vi "VCNL4010.vi"(8 "i_error":errorcluster, 10 "i_Ref":T1={"Adress"=19, "CMD"=enum."#0 Command Register", "i_Value"=0, "R/W"=enum."Read"} {"i_Value" format="%08b"; "Adress" format="%02x"}) -> (0 "o_error":errorcluster, 2 "o_data":u8 format="%x")   [LabVIEW 2016]
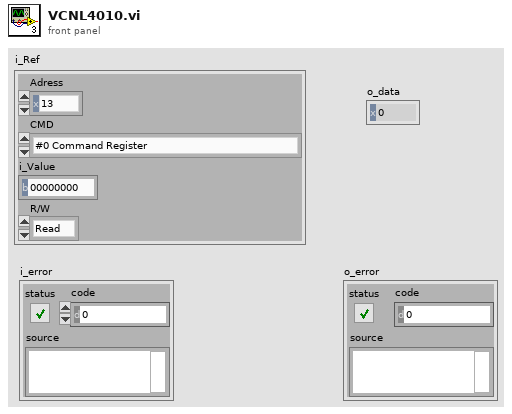
[diagram p1: front panel]
types:
  T1 = cluster{"Adress":u8, "CMD":enum8{"#0 Command Register", "#1 Product ID Revision Register", "#2 Proximity Rate Register", "#3 IR LED Current Register", "#4 Ambient Light Parameter Register", "#5 Ambient Light Result Register", "#6 Ambient Light Result Register", "#7 Proximity Result Register", "#8 Proximity Result Register", "#9 Interrupt Control Register", "#10 Low Threshold Register", "#11 Low Threshold Register", "#12 High Threshold Register", "#13 High Threshold Register", "#14 Interrupt Status Register", "#15 Proximity Modulation Timing Adjustment"}, "i_Value":u8, "R/W":enum16{"Read", "Write"}}
  T2 = enum8{"#0 Command Register", "#1 Product ID Revision Register", "#2 Proximity Rate Register", "#3 IR LED Current Register", "#4 Ambient Light Parameter Register", "#5 Ambient Light Result Register", "#6 Ambient Light Result Register", "#7 Proximity Result Register", "#8 Proximity Result Register", "#9 Interrupt Control Register", "#10 Low Threshold Register", "#11 Low Threshold Register", "#12 High Threshold Register", "#13 High Threshold Register", "#14 Interrupt Status Register", "#15 Proximity Modulation Timing Adjustment"}
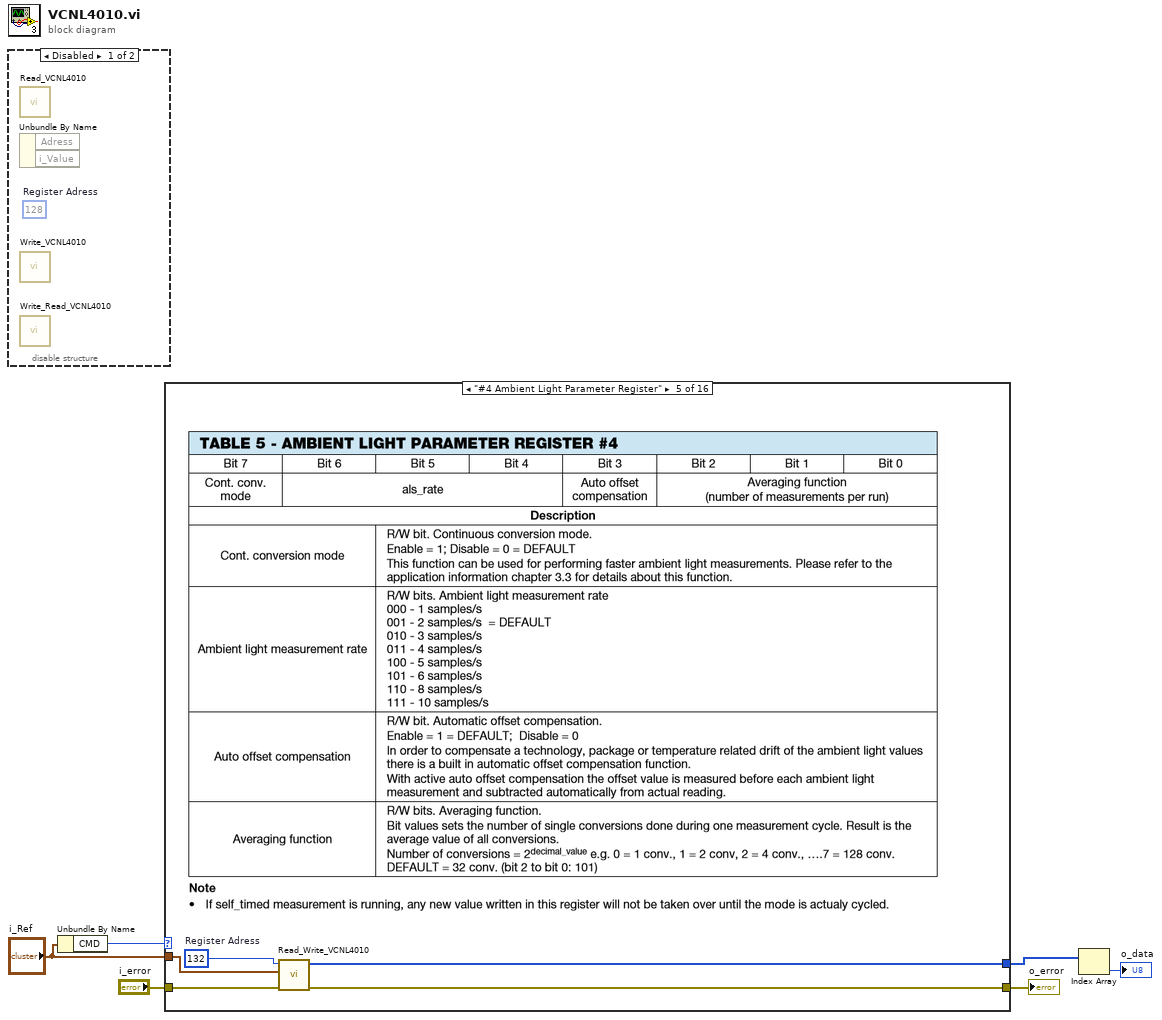
[diagram p0: block diagram]
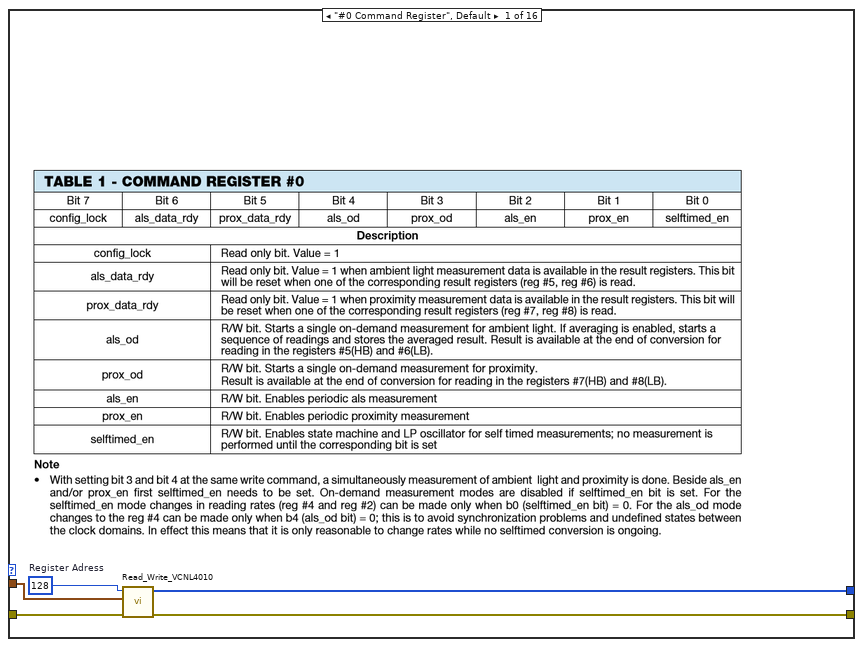
[diagram p2: hidden frame]
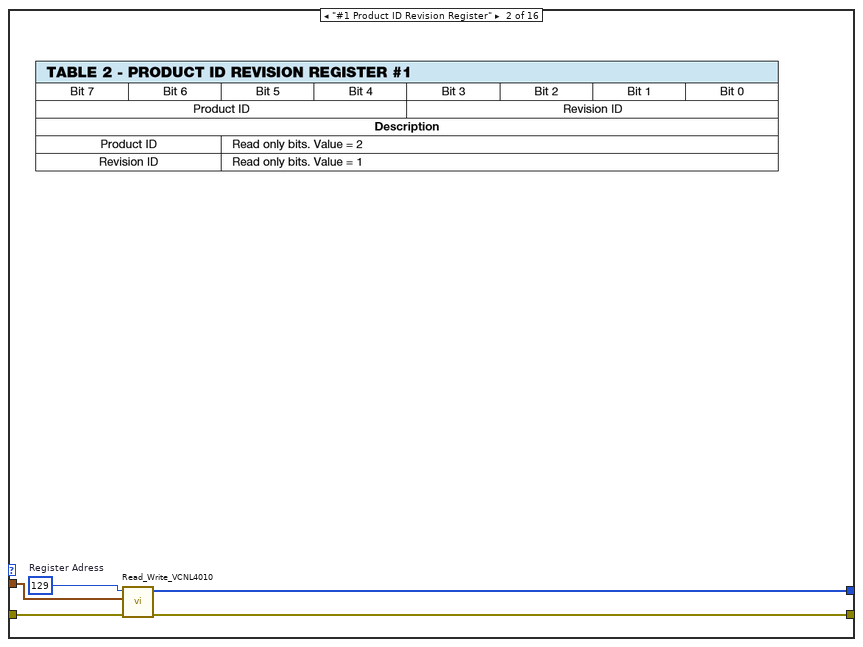
[diagram p3: hidden frame]
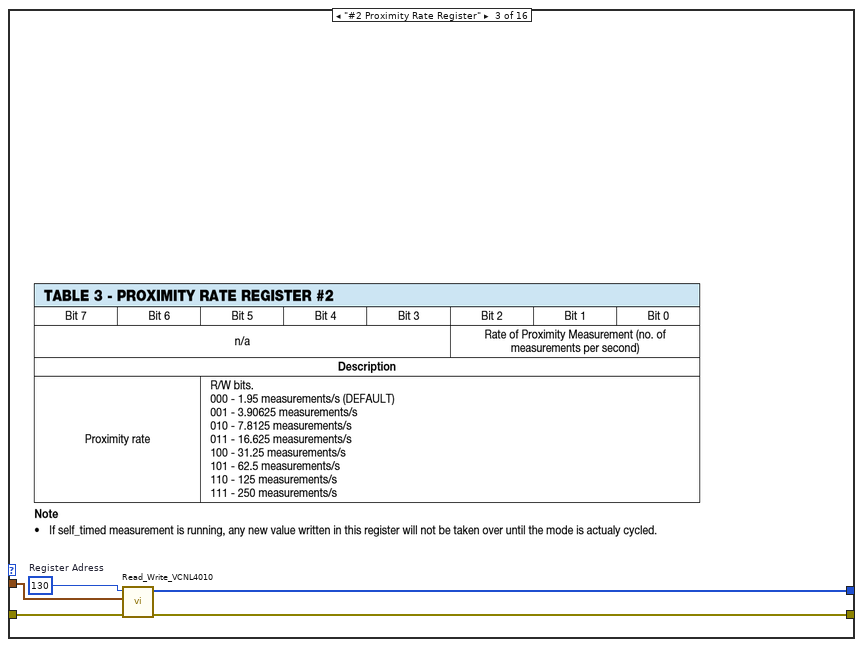
[diagram p4: hidden frame]
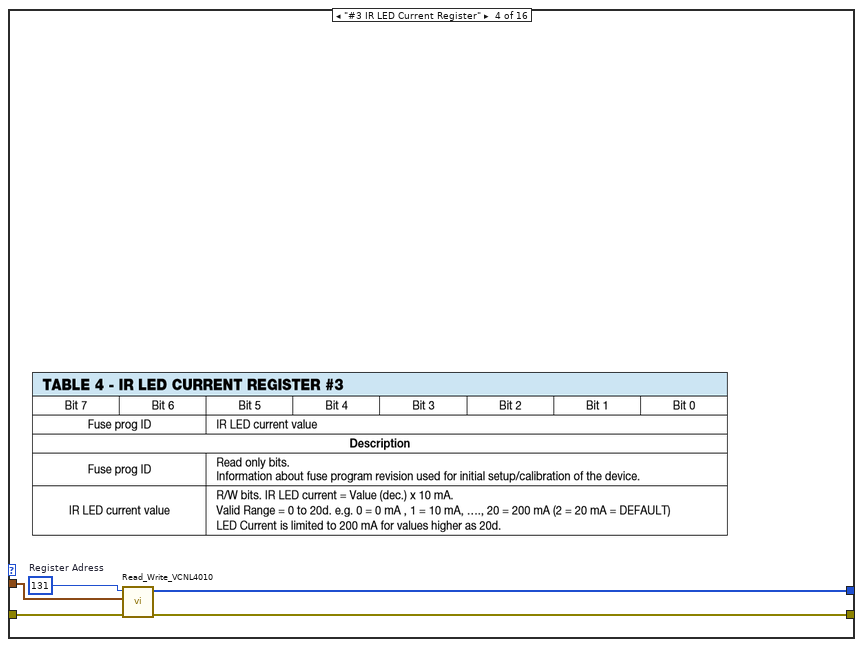
[diagram p5: hidden frame]
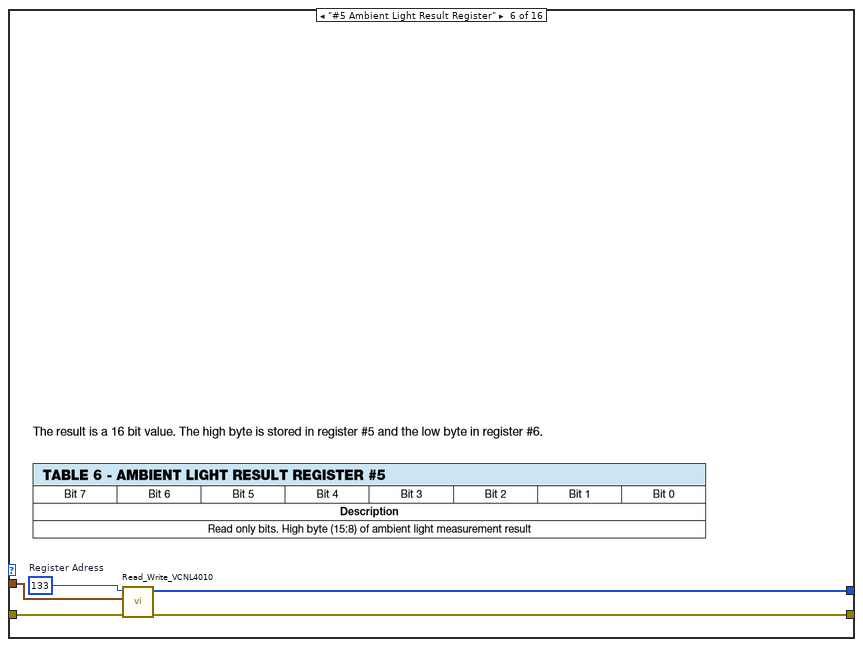
[diagram p6: hidden frame]
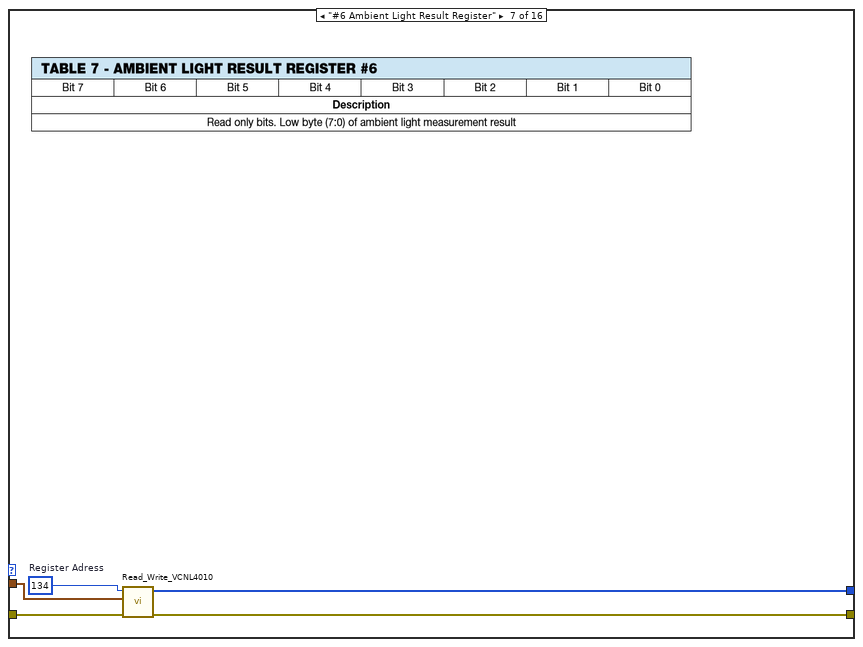
[diagram p7: hidden frame]
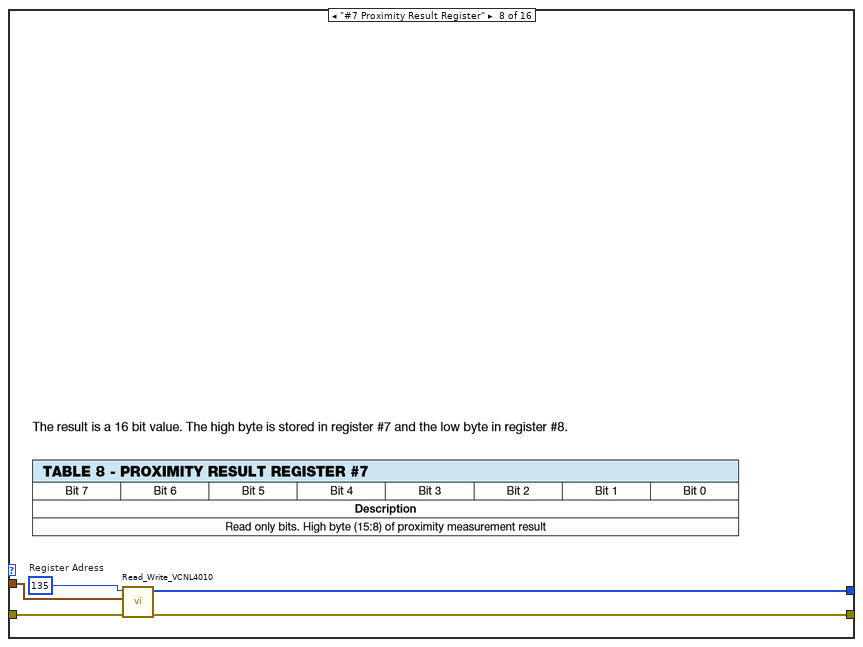
[diagram p8: hidden frame]
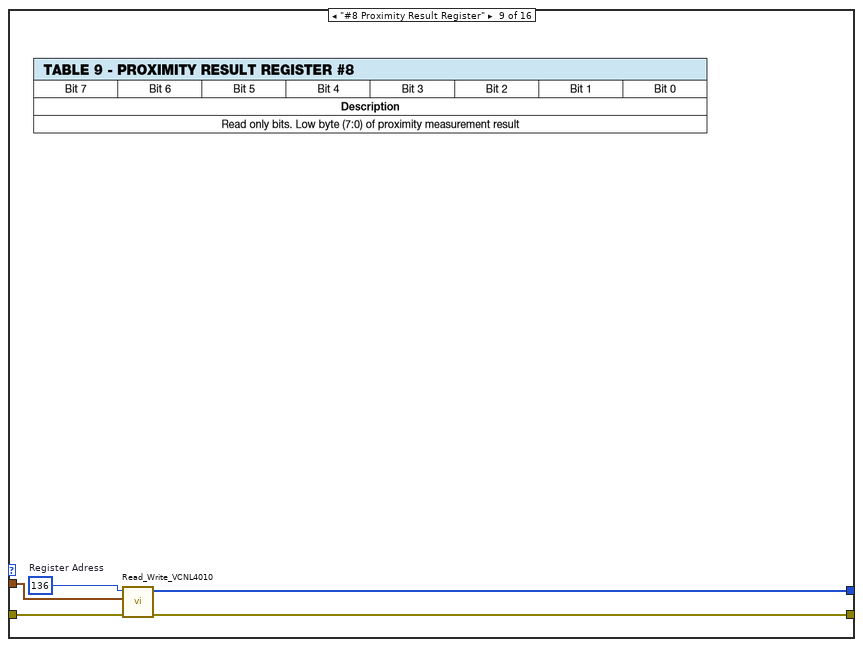
[diagram p9: hidden frame]
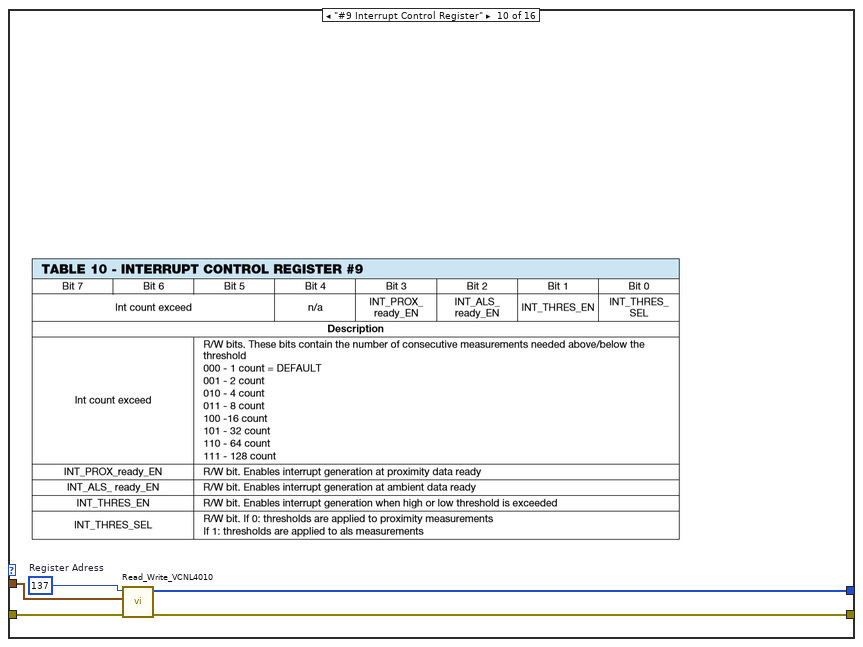
[diagram p10: hidden frame]
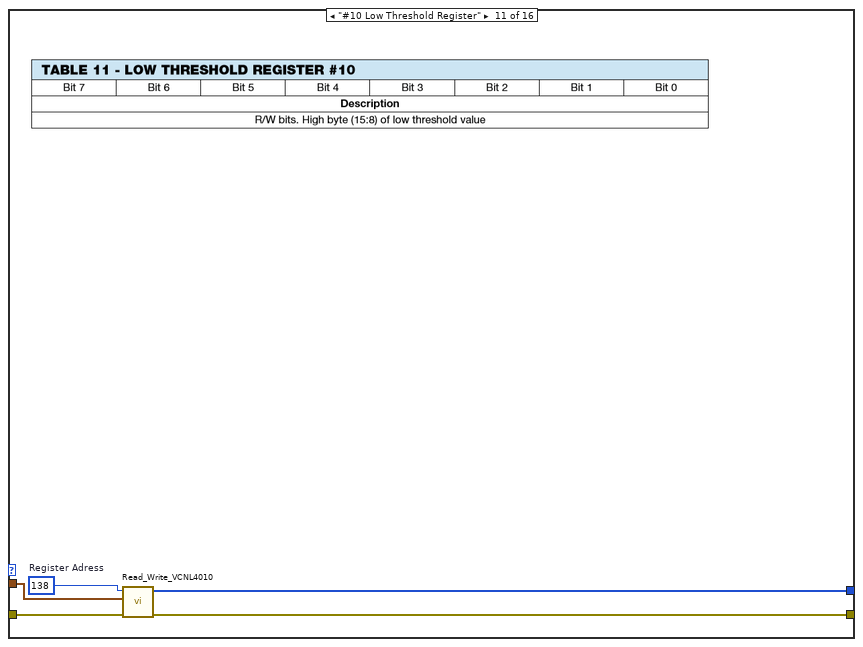
[diagram p11: hidden frame]
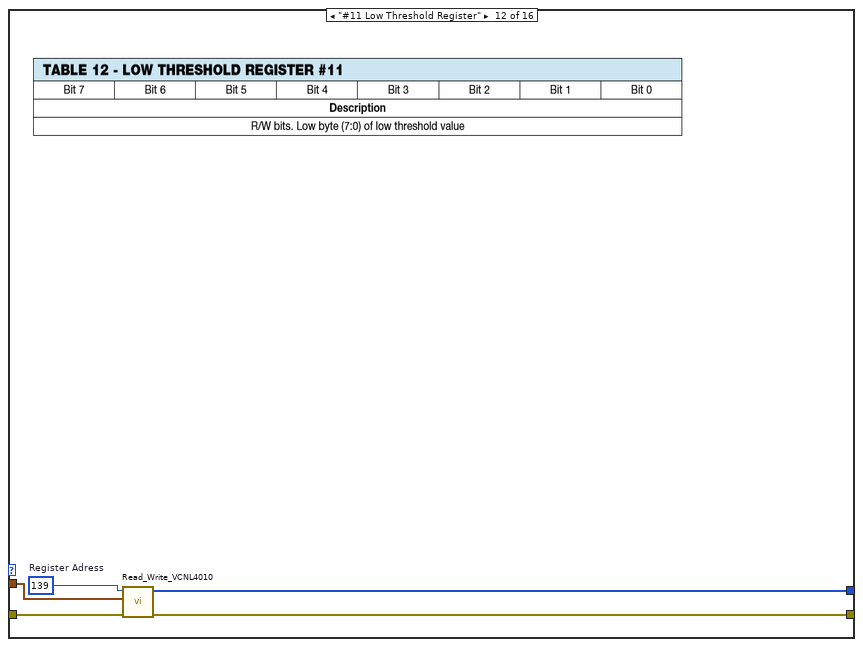
[diagram p12: hidden frame]
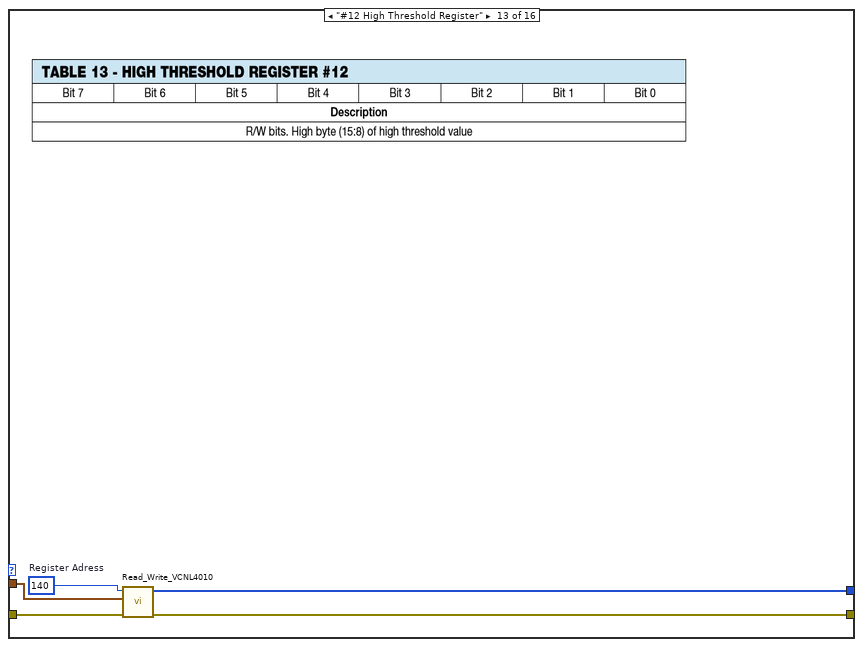
[diagram p13: hidden frame]
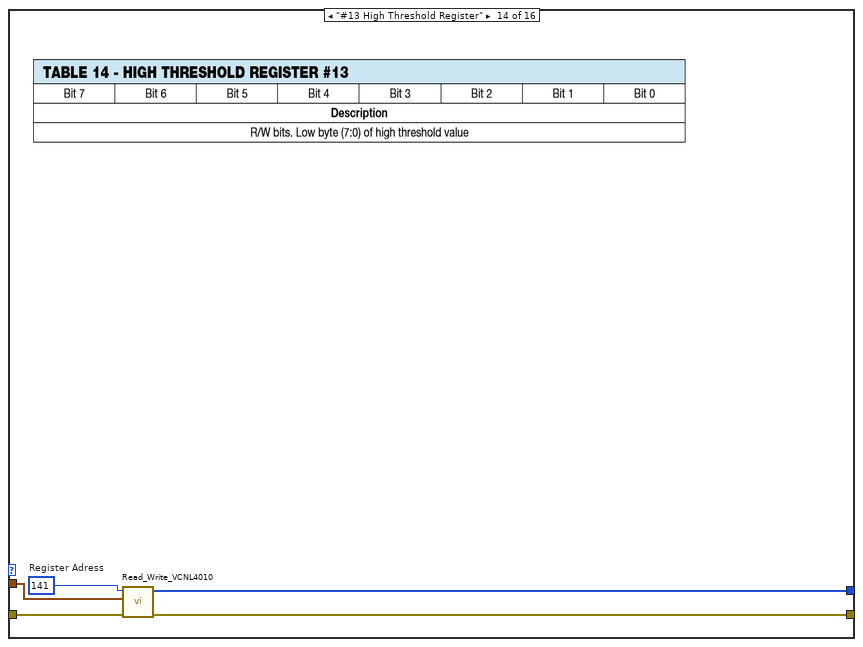
[diagram p14: hidden frame]
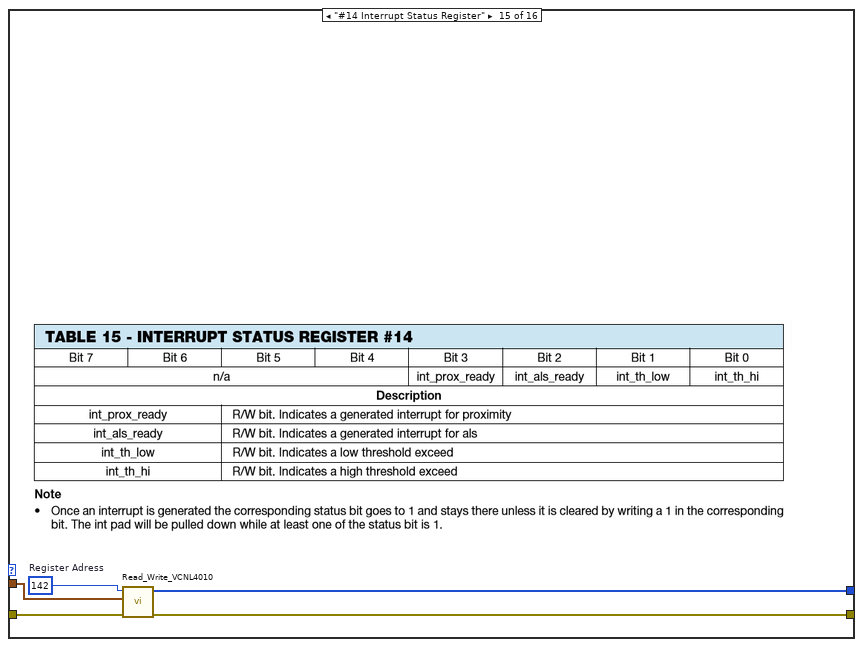
[diagram p15: hidden frame]
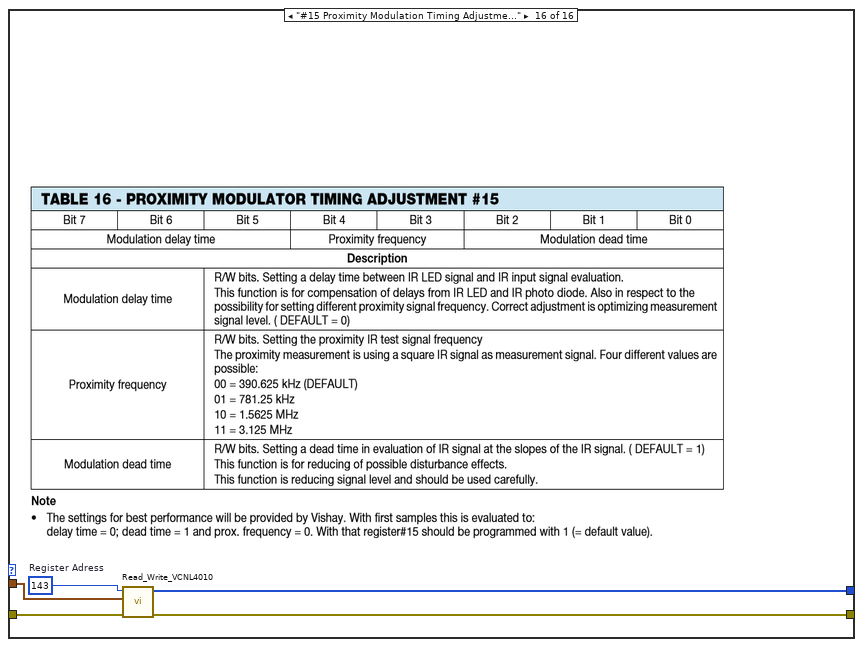
[diagram p16: hidden frame]
diagram:
  n1 = disable-structure shown="Disabled" {
    frame Disabled {
      (unwired) 128  # Register Adress
      n2 = call "Read_VCNL4010.vi"() -> ()  [unwired: 10 in, 2 out]
      n3 = Unbundle By Name() -> ()  [unwired: 1 in, 2 out]
      n4 = call "Write_VCNL4010.vi"() -> ()  [unwired: 11 in, 1 out]
      n5 = call "Write_Read_VCNL4010.vi"() -> ()  [unwired: 10 in, 2 out]
    }
    frame Enabled {
    }
  }
  n6 = Unbundle By Name("i_Ref") -> ("CMD"=w3:T2)
  n7 = case shown="\"#4 Ambient Light Parameter Register\"" w3 {
    tunnel: "i_Ref" -> [w10 w15 w20 w25 w31 w36 w41 w45 w50 w55 w60 w65 w70 w75 w80 w85]
    tunnel: [w7 w12 w17 w22 w27 w32 w38 w42 w47 w52 w57 w62 w67 w72 w77 w82] -> w2
    tunnel: "i_error" -> [w9 w14 w19 w24 w29 w34 w39 w44 w49 w54 w59 w64 w69 w74 w79 w84]
    tunnel: [w8 w13 w18 w23 w28 w33 w37 w43 w48 w53 w58 w63 w68 w73 w78 w83] -> w4
    frame "#0 Command Register", Default {
      w11 = u8 128  # Register Adress
      n8 = call "Read_Write_VCNL4010.vi"("error in (no error)"=w9, "i_Ref"=w10, "Register Adress"=w11) -> ("error out"=w8:errorcluster, "Bytes Read"=w7:u8[])  [unwired: 7 in]
    }
    frame "#1 Product ID Revision Register" {
      w16 = u8 129  # Register Adress
      n9 = call "Read_Write_VCNL4010.vi"("error in (no error)"=w14, "i_Ref"=w15, "Register Adress"=w16) -> ("error out"=w13:errorcluster, "Bytes Read"=w12:u8[])  [unwired: 7 in]
    }
    frame "#2 Proximity Rate Register" {
      w21 = u8 130  # Register Adress
      n10 = call "Read_Write_VCNL4010.vi"("error in (no error)"=w19, "i_Ref"=w20, "Register Adress"=w21) -> ("error out"=w18:errorcluster, "Bytes Read"=w17:u8[])  [unwired: 7 in]
    }
    frame "#3 IR LED Current Register" {
      w26 = u8 131  # Register Adress
      n11 = call "Read_Write_VCNL4010.vi"("error in (no error)"=w24, "i_Ref"=w25, "Register Adress"=w26) -> ("error out"=w23:errorcluster, "Bytes Read"=w22:u8[])  [unwired: 7 in]
    }
    frame "#4 Ambient Light Parameter Register" {
      w30 = u8 132  # Register Adress
      n12 = call "Read_Write_VCNL4010.vi"("error in (no error)"=w29, "i_Ref"=w31, "Register Adress"=w30) -> ("error out"=w28:errorcluster, "Bytes Read"=w27:u8[])  [unwired: 7 in]
    }
    frame "#5 Ambient Light Result Register" {
      w35 = u8 133  # Register Adress
      n13 = call "Read_Write_VCNL4010.vi"("error in (no error)"=w34, "i_Ref"=w36, "Register Adress"=w35) -> ("error out"=w33:errorcluster, "Bytes Read"=w32:u8[])  [unwired: 7 in]
    }
    frame "#6 Ambient Light Result Register" {
      w40 = u8 134  # Register Adress
      n14 = call "Read_Write_VCNL4010.vi"("error in (no error)"=w39, "i_Ref"=w41, "Register Adress"=w40) -> ("error out"=w37:errorcluster, "Bytes Read"=w38:u8[])  [unwired: 7 in]
    }
    frame "#7 Proximity Result Register" {
      w46 = u8 135  # Register Adress
      n15 = call "Read_Write_VCNL4010.vi"("error in (no error)"=w44, "i_Ref"=w45, "Register Adress"=w46) -> ("error out"=w43:errorcluster, "Bytes Read"=w42:u8[])  [unwired: 7 in]
    }
    frame "#8 Proximity Result Register" {
      w51 = u8 136  # Register Adress
      n16 = call "Read_Write_VCNL4010.vi"("error in (no error)"=w49, "i_Ref"=w50, "Register Adress"=w51) -> ("error out"=w48:errorcluster, "Bytes Read"=w47:u8[])  [unwired: 7 in]
    }
    frame "#9 Interrupt Control Register" {
      w56 = u8 137  # Register Adress
      n17 = call "Read_Write_VCNL4010.vi"("error in (no error)"=w54, "i_Ref"=w55, "Register Adress"=w56) -> ("error out"=w53:errorcluster, "Bytes Read"=w52:u8[])  [unwired: 7 in]
    }
    frame "#10 Low Threshold Register" {
      w61 = u8 138  # Register Adress
      n18 = call "Read_Write_VCNL4010.vi"("error in (no error)"=w59, "i_Ref"=w60, "Register Adress"=w61) -> ("error out"=w58:errorcluster, "Bytes Read"=w57:u8[])  [unwired: 7 in]
    }
    frame "#11 Low Threshold Register" {
      w66 = u8 139  # Register Adress
      n19 = call "Read_Write_VCNL4010.vi"("error in (no error)"=w64, "i_Ref"=w65, "Register Adress"=w66) -> ("error out"=w63:errorcluster, "Bytes Read"=w62:u8[])  [unwired: 7 in]
    }
    frame "#12 High Threshold Register" {
      w71 = u8 140  # Register Adress
      n20 = call "Read_Write_VCNL4010.vi"("error in (no error)"=w69, "i_Ref"=w70, "Register Adress"=w71) -> ("error out"=w68:errorcluster, "Bytes Read"=w67:u8[])  [unwired: 7 in]
    }
    frame "#13 High Threshold Register" {
      w76 = u8 141  # Register Adress
      n21 = call "Read_Write_VCNL4010.vi"("error in (no error)"=w74, "i_Ref"=w75, "Register Adress"=w76) -> ("error out"=w73:errorcluster, "Bytes Read"=w72:u8[])  [unwired: 7 in]
    }
    frame "#14 Interrupt Status Register" {
      w81 = u8 142  # Register Adress
      n22 = call "Read_Write_VCNL4010.vi"("error in (no error)"=w79, "i_Ref"=w80, "Register Adress"=w81) -> ("error out"=w78:errorcluster, "Bytes Read"=w77:u8[])  [unwired: 7 in]
    }
    frame "#15 Proximity Modulation Timing Adjustment" {
      w86 = u8 143  # Register Adress
      n23 = call "Read_Write_VCNL4010.vi"("error in (no error)"=w84, "i_Ref"=w85, "Register Adress"=w86) -> ("error out"=w83:errorcluster, "Bytes Read"=w82:u8[])  [unwired: 7 in]
    }
  }
  "o_error" <- w4
  n24 = Index Array(array=w2) -> (element=→"o_data":u8)  [unwired: 1 in]
